vi "ret vs volt.vi"() -> ()   [LabVIEW 2014]
uses:
  <vilib>/Utility/file.llb/Write To Spreadsheet File (DBL).vi
  <vilib>/Analysis/NI_AALBase.lvlib
panel:
  out "min beam":dbl[](array[numeric])
  in  "LCVR temp":sgl=30.0 min=10 max=50
  out "max beam":dbl[](array[numeric])
  in  "Start calibration":bool
  out "Intensity Graph":dbl[][](graph)
  out "Horizontal ?":bool
  in  "OK":bool
  out "X - centroid":dbl[](array[numeric])
  out "Y - centroid":dbl[](array[numeric])
  in  "OpenStructureIn":T1={"Size"=88, "InterfaceType"=1, "Camera Number"=0, "CameraNumAtInterface"=0, "OpenFlags"=[], "OpenDWFlags"=[], "OpenPtrs"=[]} {"InterfaceType" items=["IEEE1394/FireWire", "IEEE1394/FireWire", "Matrox Helios CameraLink", "SiliconSoftware MicroEnableIII CL", "National Instruments CameraLink", "Gigabit Ethernet", "USB", "SiliconSoftware MicroEnable IV CL", "Reserved", "Reserved", "Generic CameraLink with CLSER.DLL"]}
  in  "Exposure in msec":u32
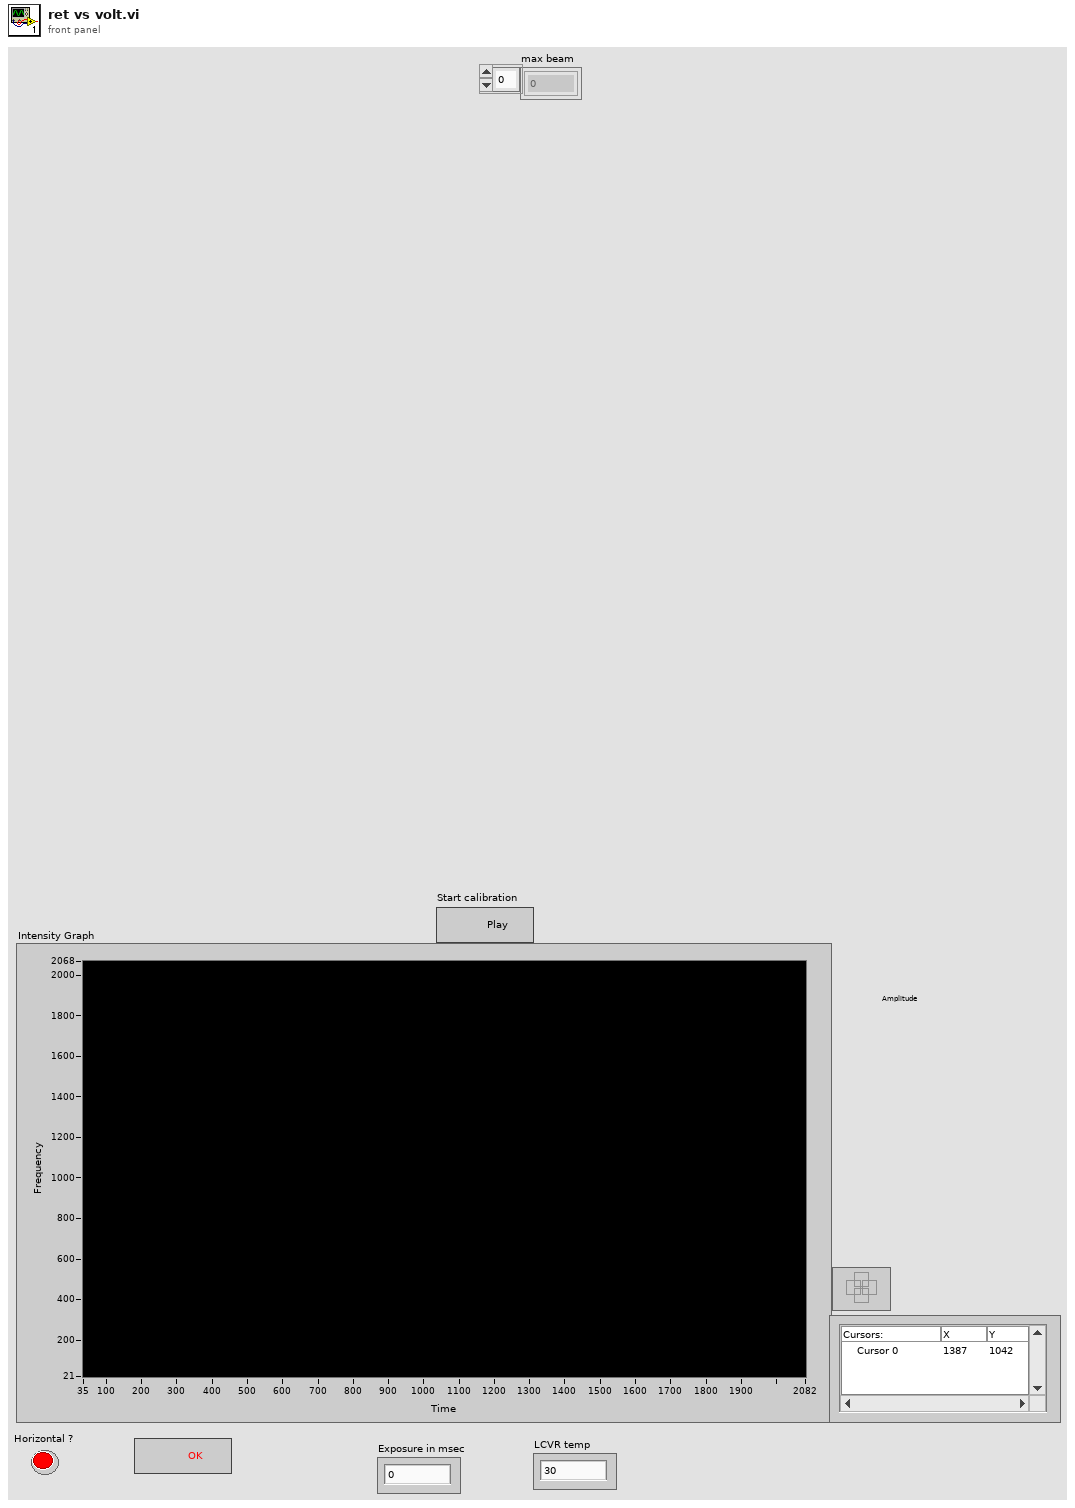
[diagram p1: front panel]
types:
  T1 = cluster{"Size":u16, "InterfaceType":u16, "Camera Number":u16, "CameraNumAtInterface":u16, "OpenFlags":u16[], "OpenDWFlags":u32[], "OpenPtrs":u32[]}
  T2 = cluster{"Device Handle":u32, "Pipe 0 Handle":u32, "Pipe 1 Handle":u32}[]
  T3 = cluster{"Device Handle":u32, "Pipe 0 Handle":u32, "Pipe 1 Handle":u32}
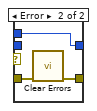
[diagram p2: hidden frame]
diagram:
  n1 = flat-sequence {
    tunnel: [w67] -> w58
    tunnel: [w66] -> w56
    tunnel: w58 -> [w112]
    tunnel: [w112] -> w57
    tunnel: w56 -> [w111]
    tunnel: [w111] -> w55
    tunnel: [w106] -> w28
    tunnel: w57 -> [w117]
    tunnel: w55 -> [w116]
    tunnel: [w114] -> w54
    tunnel: [w115] -> w52
    tunnel: w28 -> [w113]
    tunnel: [w113] -> w23
    tunnel: w54 -> [w173]
    tunnel: [w173] -> w53
    tunnel: w52 -> [w172]
    tunnel: [w172] -> w51
    tunnel: [w170] -> w24
    tunnel: w23 -> [w170]
    tunnel: w53 -> [w189]
    tunnel: w51 -> [w190]
    tunnel: [w183] -> w50
    tunnel: [w187] -> w47
    tunnel: [w186] -> w45
    tunnel: [w185] -> w41
    tunnel: [w184] -> w38
    tunnel: w29 -> [w183]
    tunnel: [w182] -> w25
    tunnel: w24 -> [w182]
    tunnel: [w176] -> w22
    tunnel: w50 -> [w253]
    tunnel: [w253] -> w49
    tunnel: [w250] -> w48
    tunnel: w47 -> [w250]
    tunnel: [w249] -> w46
    tunnel: w45 -> [w249]
    tunnel: [w248] -> w42
    tunnel: w41 -> [w248]
    tunnel: [w247] -> w39
    tunnel: w38 -> [w247]
    tunnel: [w246] -> w26
    tunnel: w25 -> [w246]
    tunnel: w22 -> [w245]
    tunnel: [w245] -> w20
    tunnel: w49 -> [w261]
    tunnel: [w261] -> w44
    tunnel: w48 -> [w255]
    tunnel: w46 -> [w257]
    tunnel: [w259] -> w43
    tunnel: w42 -> [w259]
    tunnel: [w258] -> w40
    tunnel: w39 -> [w258]
    tunnel: [w257] -> w35
    tunnel: [w256] -> w27
    tunnel: w26 -> [w256]
    tunnel: [w255] -> w21
    tunnel: w20 -> [w254]
    tunnel: [w254] -> w19
    tunnel: w44 -> [w265]
    tunnel: [w265] -> w18
    tunnel: w43 -> [w262]
    tunnel: w40 -> [w271]
    tunnel: [w270] -> w17
    tunnel: [w269] -> w16
    tunnel: [w268] -> w15
    tunnel: w35 -> [w268]
    tunnel: w27 -> [w267]
    tunnel: w21 -> [w264]
    tunnel: w19 -> [w263]
    tunnel: w18 -> [w327]
    tunnel: [w327] -> w14
    tunnel: w17 -> [w326]
    tunnel: [w326] -> w13
    tunnel: w16 -> [w325]
    tunnel: [w325] -> w12
    tunnel: w15 -> [w324]
    tunnel: [w324] -> w11
    tunnel: w14 -> [w337]
    tunnel: [w337] -> w10
    tunnel: w13 -> [w332]
    tunnel: [w330] -> w8
    tunnel: w12 -> [w333]
    tunnel: [w331] -> w6
    tunnel: w11 -> [w336]
    tunnel: [w336] -> w4
    tunnel: [w328] -> w2
    tunnel: w10 -> [w344]
    tunnel: [w344] -> w9
    tunnel: w8 -> [w343]
    tunnel: [w343] -> w7
    tunnel: w6 -> [w342]
    tunnel: [w342] -> w5
    tunnel: w4 -> [w341]
    tunnel: [w341] -> w3
    tunnel: w2 -> [w340]
    tunnel: [w340] -> w1
    tunnel: w9 -> [w357]
    tunnel: w7 -> [w352]
    tunnel: w5 -> [w351]
    tunnel: [w349] -> w37
    tunnel: [w348] -> w36
    tunnel: w3 -> [w348]
    tunnel: [w347] -> w34
    tunnel: [w346] -> w33
    tunnel: w1 -> [w345]
    tunnel: w37 -> [w412]
    tunnel: w36 -> [w427]
    tunnel: w34 -> [w418]
    tunnel: w33 -> [w417]
    frame #0 {
      w70 = u16 1 items=["Stop", "Run"] ("RecordingState")
      w73 = u16 1 items=["Auto", "Software", "External sequence start ", "External exposure control"] ("TriggerMode")
      w82 = u16 2 items=["nanoseconds", "microseconds", "milliseconds"] ("ExposureTimeBase")
      w61 = u32 8388608 ("Size")
      w92 = u16 0 items=["Stop", "Run"] ("RecordingState")
      n2 = local read "OpenStructureIn"() -> (w100:T1)
      n3 = Bundle By Name(cluster=w100, "InterfaceType"=u16 6) -> (w98:T1)
      n4 = call <userlib>:"OpenCameraEx.vi"("OpenStructureIn"=w98) -> ("error out"=w96:errorcluster, "hout"=w97:u64)  [unwired: 3 in, 2 out]
      n5 = call <userlib>:"CancelImages.vi"("error in (no error)"=w96, "ph"=w97) -> ()  [unwired: 1 in, 3 out]
      n6 = call <userlib>:"InitLibrary.vi"("error in (no error)"=w96, "InterfaceType"=u32 3, "ph"=w97) -> ("error out"=w93:errorcluster, "hout"=w94:u64)  [unwired: 7 in]
      n7 = call <userlib>:"SetBitAlignment.vi"("error in (no error)"=w93, "BitAlignent"=TRUE, "ph"=w94) -> ("error out"=w72:errorcluster, "hout"=w77:u64)  [unwired: 2 in, 1 out]
      n8 = call <userlib>:"SetStorageMode.vi"("error in (no error)"=w72, "StorageMode"=TRUE, "ph"=w77) -> ("error out"=w74:errorcluster, "hout"=w75:u64)  [unwired: 2 in, 1 out]
      n9 = call <userlib>:"SetTrigger.vi"("error in (no error)"=w74, "TriggerMode"=w73, "ph"=w75) -> ("error out"=w64:errorcluster, "hout"=w65:u64)  [unwired: 2 in, 1 out]
      n10 = call <userlib>:"AllocateBuffer.vi"("error in (no error)"=w64, "Size"=w61, "BufNr"=i16 -1, "ph"=w65) -> ("error out"=w63:errorcluster, "BufNrOut"=w59:i16, "hout"=w62:u64)  [unwired: 2 in, 3 out]
      n11 = call <userlib>:"SetRecordingState.vi"("ErrorIn"=w63, "RecordingState"=w92, "ph"=w62) -> ("ErrorOut"=w90:errorcluster, "hout"=w91:u64)  [unwired: 2 in, 1 out]
      n12 = case shown="No Error" w90 {
        tunnel: [w102 w104] -> w88
        tunnel: w90 -> [w102 w105]
        tunnel: w91 -> [w101 _]
        tunnel: [w101 w103] -> w89
        tunnel: w77 -> [_ w103]
        frame No Error {
        }
        frame Error {
          n13 = call <vilib>:"Clear Errors.vi"("error in (no error)"=w105) -> ("error out"=w104:errorcluster)  [unwired: 5 in, 1 out]
        }
      }
      n14 = call <userlib>:"AllocateBuffer.vi"("error in (no error)"=w88, "Size"=w61, "BufNr"=i16 -1, "ph"=w89) -> ("error out"=w85:errorcluster, "hout"=w86:u64)  [unwired: 2 in, 4 out]
      n15 = call <userlib>:"SetDelayExposureTime.vi"("ph"=w86, "Delay"=u32 0, "Exposure"="Exposure in msec", "error in (no error)"=w85, "DelayTimeBase"=w82, "ExposureTimeBase"=w82) -> ("hout"=w81:u64, "error out"=w80:errorcluster)  [unwired: 7 in, 1 out]
      n16 = call <userlib>:"ArmCamera.vi"("error in (no error)"=w80, "ph"=w81) -> ("error out"=w78:errorcluster, "hout"=w79:u64)  [unwired: 2 out]
      n17 = call <userlib>:"AllocateBuffer.vi"("error in (no error)"=w78, "Size"=w61, "BufNr"=w59, "ph"=w79) -> ("error out"=w68:errorcluster, "hout"=w71:u64)  [unwired: 2 in, 4 out]
      n18 = call <userlib>:"SetRecordingState.vi"("ErrorIn"=w68, "RecordingState"=w70, "ph"=w71) -> ("ErrorOut"=w66:errorcluster, "hout"=w67:u64)  [unwired: 2 in, 1 out]
    }
    frame #1 {
      n19 = One Button Dialog(message="After starting and making the beam\nhorizintal cross one of the beam with\npolariser place lcvr and then press OK\n button to initiate voltage vs ret \n   calibration              ", button name ("OK")="Got it !!") -> ()  [unwired: 1 out]
      n20 = call "File Dialog3"("prompt"="Select folder containing matlab files for execution") -> ("selected path"=w107:path)  [unwired: 11 in, 3 out]
      n21 = Path To String(path=w107) -> (string=w106:string)
    }
    frame #2 {
      # "To check if  beams of beam splitter are perfectly horizontal"
      n22 = while {
        tunnel: ["Start calibration"] -> w118
        stop <- "Start calibration" stop-if-true
      }
      n23 = while {
        shift-right: [w125] -> w115
        shift-left: w117 -> [w131]
        shift-right: [w124] -> w114
        shift-left: w116 -> [w130]
        stop <- w120 stop-if-true
        n24 = call <userlib>:"ForceTrigger.vi"("ph"=w131, "error in (no error)"=w130) -> ("hout"=w129:u64, "error out"=w128:errorcluster)  [unwired: 1 in, 2 out]
        n25 = call "grab image_2.vi"("ErrorIn"=w128, "Image number"=u32 0, "BuffNr"=i16 0, "ph"=w129) -> ("output image"=→"Intensity Graph":dbl[][], "error out"=w124:errorcluster, "Buffer_Ready"=w121:bool, "hout"=w125:u64)  [unwired: 4 in]
        n26 = local read "OK"() -> (w122:bool)
        n27 = And(x=w121, y=w122) -> (x .and. y?=w120:bool)
      }
      n28 = case shown="True" w118 {
        tunnel: w113 -> [_ w132]
        frame False {
        }
        frame True {
          n29 = while {
            tunnel: w132 -> [w134]
            stop <- w133 stop-if-true
            n30 = flat-sequence {
              tunnel: w134 -> [w141]
              tunnel: [w151] -> w133
              frame #0 {
                n31 = local read "Intensity Graph"() -> (w135:dbl[][])
                n32 = property on="Intensity Graph" class="IntGraph (strict)"() -> ("Cursor.Cursor X"=w142:dbl)  [unwired: 2 in, 2 out]
                n33 = script code="cd(path);\n[ax,ay]=calib1(da,s);\nx=[ax(1),ay(1)];\ny=[ax(2),ay(2)];"("path"=w141, "da"=w135, "s"=w142) -> ("x"=w140:dbl[], "y"=w139:dbl[])  [unwired: 1 in, 1 out]
                "X - centroid" <- w140
                "Y - centroid" <- w139
                n34 = Reshape Array(w135, 4194304 ("dimension size")) -> (w143:dbl[])
                n35 = call <vilib>:"Median.vi"("X"=w143) -> ("median"=w138:dbl)  [unwired: 1 out]
                n36 = Index Array(array=w140, index=1) -> (element=w148:dbl)
                n37 = Index Array(array=w139, index=1) -> (element=w147:dbl)
                n38 = call "= to within Tolerance"("Operand 2"=w147, "Operand 1"=w148) -> ("Result"=w146:dynamicdata)  [unwired: 8 in, 1 out]
                n39 = Add(x=w138, y=700.0) -> (x+y=w136:dbl)
                n40 = call "Convert from Dynamic Data"("Dynamic Data Type"=w146) -> ("Scalar"=→"Horizontal ?":bool)  [unwired: 3 in]
                n41 = property on="Intensity Graph" class="IntGraph (strict)"("ZScale.Maximum"=w136) -> ()  [unwired: 2 in, 2 out]
              }
              frame #1 {
                n42 = Two Button Dialog(message="repeat curve \n  fit?         ", 1:"yes" ("F button name (\"Cancel\")"), 2:"no" ("T button name (\"OK\")")) -> (T button?=w151:bool)
                n43 = local write "OK"(w151) -> ()
              }
            }
          }
        }
      }
    }
    frame #3 {
      n44 = local read "X - centroid"() -> (w162:dbl[])
      n45 = local read "Y - centroid"() -> (w161:dbl[])
      n46 = local write "OK"(FALSE ("OK")) -> ()
      n47 = local read "Intensity Graph"() -> (w171:dbl[][])
      n48 = call "Convert to Dynamic Data3"("Array"=w161) -> ("Dynamic Data Type"=w160:dynamicdata)  [unwired: 3 in]
      n49 = call "Convert to Dynamic Data2"("Array"=w162) -> ("Dynamic Data Type"=w157:dynamicdata)  [unwired: 3 in]
      n50 = call "Convert from Dynamic Data3"("Dynamic Data Type"=w160) -> ("Scalar"=w159:dbl)  [unwired: 3 in]
      n51 = call "Convert from Dynamic Data4"("Dynamic Data Type"=w160) -> ("Scalar"=w158:dbl)  [unwired: 3 in]
      n52 = call "Convert from Dynamic Data5"("Dynamic Data Type"=w157) -> ("Scalar"=w156:dbl)  [unwired: 3 in]
      n53 = call "Convert from Dynamic Data6"("Dynamic Data Type"=w157) -> ("Scalar"=w155:dbl)  [unwired: 3 in]
      n54 = Index Array(array=w171, index (row)=w159, index (col)=w158) -> (element=w164:dbl)
      n55 = Index Array(array=w171, index (row)=w156, index (col)=w155) -> (element=w165:dbl)
      n56 = Greater?(x=w164, y=w165) -> (0:w163:bool)
      n57 = Greater?(x=w165, y=w164) -> (0:w168:bool)
      n58 = Select(t=w162, s=w163, f=w161) -> (s? t:f=→"min beam":dbl[])
      n59 = Select(t=w162, s=w168, f=w161) -> (s? t:f=→"max beam":dbl[])
    }
    frame #4 {
      w181 = dbl[] []
      # "to get beams of nearly equal intensity\nfor curve fitting in matlab. Note this \nvoltage neednot correspond to 90deg\nnor might it give good intensity values \nfor curve fit after aligning the lcvr"
      # "to get volt corresponding to 180deg ret"
      n60 = call "version.vi"("USB Open Device Cluster"=w183) -> ("Version"=w187:dbl)  [unwired: 10 in]
      n61 = for {
        N: 100 -> [_]
        tunnel: w183 -> [w208]
        shift-right: [w205] -> w177
        shift-left: w181 -> [w206]
        shift-right: [w203] -> w185
        shift-left: w190 -> [w204]
        shift-right: [w201] -> w184
        shift-left: w189 -> [w202]
        shift-right: [w200] -> w180
        shift-left: w181 -> [w199]
        tunnel: w187 -> [w194]
        shift-right: [w193] -> w179
        shift-left: w181 -> [w192]
        i -> [w207]
        n62 = flat-sequence {
          tunnel: w208 -> [w239]
          tunnel: w207 -> [w237]
          tunnel: w206 -> [w234]
          tunnel: w204 -> [w228]
          tunnel: w202 -> [w226]
          tunnel: w199 -> [w221]
          tunnel: [w233] -> w198
          tunnel: [w227] -> w197
          tunnel: [w225] -> w196
          tunnel: [w222] -> w195
          tunnel: w194 -> [w220]
          tunnel: [w216] -> w193
          tunnel: w192 -> [w215]
          tunnel: [w241] -> w200
          tunnel: [w242] -> w201
          tunnel: [w243] -> w203
          tunnel: [w244] -> w205
          tunnel: w198 -> [w244]
          tunnel: w197 -> [w243]
          tunnel: w196 -> [w242]
          tunnel: w195 -> [w241]
          frame #0 {
            n63 = call <userlib>:"ForceTrigger.vi"("ph"=w228, "error in (no error)"=w226) -> ("hout"=w232:u64, "error out"=w231:errorcluster)  [unwired: 1 in, 2 out]
            n64 = Divide(x=w237, y=10) -> (x/y=w235:dbl)
            n65 = local read "max beam"() -> (w224:dbl[])
            n66 = local read "min beam"() -> (w219:dbl[])
            n67 = call "Meadowlark USB Set Voltage.VI"("LC Voltage"=w235, "LC Channel"=1, "FW Version"=w220, "USB Open Device Cluster"=w239) -> ()  [unwired: 1 out]
            n68 = Build Array (concatenate)(w234, w235) -> (w233:dbl[])
            n69 = call "grab image_2.vi"("ErrorIn"=w231, "Image number"=u32 0, "BuffNr"=i16 0, "ph"=w232) -> ("output image"=w218:dbl[][], "error out"=w225:errorcluster, "hout"=w227:u64)  [unwired: 4 in, 1 out]
            n70 = call "Convert to Dynamic Data6"("Array"=w219) -> ("Dynamic Data Type"=w214:dynamicdata)  [unwired: 3 in]
            n71 = call "Convert to Dynamic Data"("Array"=w224) -> ("Dynamic Data Type"=w211:dynamicdata)  [unwired: 3 in]
            n72 = local write "Intensity Graph"(w218) -> ()
            n73 = call "Convert from Dynamic Data7"("Dynamic Data Type"=w214) -> ("Scalar"=w213:dbl)  [unwired: 3 in]
            n74 = call "Convert from Dynamic Data8"("Dynamic Data Type"=w214) -> ("Scalar"=w212:dbl)  [unwired: 3 in]
            n75 = call "Convert from Dynamic Data9"("Dynamic Data Type"=w211) -> ("Scalar"=w210:dbl)  [unwired: 3 in]
            n76 = call "Convert from Dynamic Data10"("Dynamic Data Type"=w211) -> ("Scalar"=w209:dbl)  [unwired: 3 in]
            n77 = Index Array(array=w218, index (row)=w213, index (col)=w212) -> (element=w217:dbl)
            n78 = Index Array(array=w218, index (row)=w210, index (col)=w209) -> (element=w223:dbl)
            n79 = Build Array (concatenate)(w221, w223) -> (w222:dbl[])
            n80 = Build Array (concatenate)(w215, w217) -> (w216:dbl[])
          }
          frame #1 {
            n81 = Wait (ms)(milliseconds to wait=u32 30) -> ()  [unwired: 1 out]
          }
        }
      }
      n82 = Subtract(x=w180, y=w179) -> (x-y=w175:dbl[])
      n83 = Array Max & Min(array=w180) -> (min index (indices)=w188:i32)  [unwired: 3 out]
      n84 = Absolute Value(x=w175) -> (abs(x)=w174:dbl[])
      n85 = Index Array(array=w177, index=w188) -> (element=w186:dbl)
      n86 = Array Max & Min(array=w174) -> (min index (indices)=w178:i32)  [unwired: 3 out]
      n87 = Index Array(array=w177, index=w178) -> (element=w176:dbl)
    }
    frame #5 {
      n88 = One Button Dialog(message="current retardance of lcvr \nis 180deg rotate lcvr to get\nthe beam which was crossed \nto maximum intensity then \nselect the split point on the \nimage using cursor and click OK. \nThis calculates the new position \nof the two beams.       ", button name ("OK")="Yes") -> ()  [unwired: 1 out]
    }
    frame #6 {
      n89 = call "Meadowlark USB Set Voltage.VI"("LC Voltage"=w257, "LC Channel"=1, "FW Version"=w255, "USB Open Device Cluster"=w261) -> ()  [unwired: 1 out]
    }
    frame #7 {
      n90 = flat-sequence {
        tunnel: w267 -> [w272]
        tunnel: [w272] -> w266
        tunnel: w266 -> [w283]
        tunnel: w265 -> [w278]
        tunnel: w264 -> [w277]
        tunnel: w263 -> [w275]
        tunnel: w262 -> [w274]
        frame #0 {
          n91 = while {
            stop <- w273 stop-if-true
            n92 = local read "OK"() -> (w273:bool)
          }
        }
        frame #1 {
          n93 = call "Meadowlark USB Set Voltage.VI"("LC Voltage"=w275, "LC Channel"=1, "FW Version"=w277, "USB Open Device Cluster"=w278) -> ()  [unwired: 1 out]
          n94 = Two Button Dialog(message="Recalibrate position\nof the beams?  ", 1:"No" ("F button name (\"Cancel\")"), 2:"Yes" ("T button name (\"OK\")")) -> (T button?=w279:bool)
          n95 = case shown="True" w279 {
            tunnel: w283 -> [_ w287]
            tunnel: w274 -> [_ w284]
            frame False {
            }
            frame True {
              n96 = flat-sequence {
                tunnel: w287 -> [w290]
                tunnel: [w290] -> w286
                tunnel: [w289] -> w285
                tunnel: w284 -> [w288]
                tunnel: w286 -> [w303]
                tunnel: w285 -> [w299]
                frame #0 {
                  n97 = while {
                    shift-right: [w293] -> _
                    shift-left: w288 -> [w292]
                    tunnel: [w291] -> w289
                    stop <- w298 stop-if-true
                    n98 = call <userlib>:"ForceTrigger.vi"("ph"=w292) -> ("hout"=w297:u64, "error out"=w294:errorcluster)  [unwired: 2 in, 2 out]
                    n99 = call "grab image_2.vi"("ErrorIn"=w294, "Image number"=u32 0, "BuffNr"=i16 0, "ph"=w297) -> ("output image"=w291:dbl[][], "hout"=w293:u64)  [unwired: 4 in, 2 out]
                    n100 = local write "Intensity Graph"(w291) -> ()
                    n101 = local read "OK"() -> (w298:bool)
                  }
                }
                frame #1 {
                  n102 = property on="Intensity Graph" class="IntGraph (strict)"() -> ("Cursor.Cursor X"=w302:dbl)  [unwired: 2 in, 2 out]
                  n103 = script code="cd(path);\n[ax,ay]=calib1(da,s);\nx=[ax(1),ay(1)];\ny=[ax(2),ay(2)];"("path"=w303, "da"=w299, "s"=w302) -> ("x"=w301:dbl[], "y"=w300:dbl[])  [unwired: 1 in, 1 out]
                  n104 = local write "X - centroid"(w301) -> ()
                  n105 = local write "Y - centroid"(w300) -> ()
                  n106 = Index Array(array=w301, index=1) -> (element=w307:dbl)
                  n107 = Index Array(array=w300, index=1) -> (element=w306:dbl)
                  n108 = call "= to within Tolerance2"("Operand 2"=w306, "Operand 1"=w307) -> ("Result"=w305:dynamicdata)  [unwired: 8 in, 1 out]
                  n109 = call "Convert from Dynamic Data2"("Dynamic Data Type"=w305) -> ("Scalar"=w304:bool)  [unwired: 3 in]
                  n110 = local write "Horizontal ?"(w304) -> ()
                }
              }
            }
          }
        }
      }
      n111 = while {
        shift-right: [w315] -> w270
        shift-left: w262 -> [w321]
        shift-right: [w314] -> w269
        shift-left: w271 -> [w320]
        stop <- w311 stop-if-true
        n112 = call <userlib>:"ForceTrigger.vi"("ph"=w321, "error in (no error)"=w320) -> ("hout"=w319:u64, "error out"=w318:errorcluster)  [unwired: 1 in, 2 out]
        n113 = call "grab image_2.vi"("ErrorIn"=w318, "Image number"=u32 0, "BuffNr"=i16 0, "ph"=w319) -> ("output image"=w310:dbl[][], "error out"=w314:errorcluster, "Buffer_Ready"=w312:bool, "hout"=w315:u64)  [unwired: 4 in]
        n114 = local read "OK"() -> (w313:bool)
        n115 = local write "Intensity Graph"(w310) -> ()
        n116 = And(x=w312, y=w313) -> (x .and. y?=w311:bool)
      }
    }
    frame #8 {
      n117 = One Button Dialog(message="Now we will record background so \nswitch off the source and prees \nOK button                ", button name ("OK")="OK") -> ()  [unwired: 1 out]
    }
    frame #9 {
      w329 = i16 0 ("BuffNr")
      n118 = call <userlib>:"ForceTrigger.vi"("ph"=w332, "error in (no error)"=w333) -> ("hout"=w335:u64, "error out"=w334:errorcluster)  [unwired: 1 in, 2 out]
      n119 = call "grab image_2.vi"("ErrorIn"=w334, "Image number"=w329, "BuffNr"=w329, "ph"=w335) -> ("output image"=w328:dbl[][], "error out"=w331:errorcluster, "hout"=w330:u64)  [unwired: 4 in, 1 out]
      n120 = local write "Intensity Graph"(w328) -> ()
    }
    frame #10 {
      n121 = One Button Dialog(message="Switch on source\nto perform volt vs\nret calibration and\npress OK     ", button name ("OK")="OK") -> ()  [unwired: 1 out]
    }
    frame #11 {
      w350 = dbl[] []
      n122 = call "version.vi"("USB Open Device Cluster"=w357) -> ("Version"=w356:dbl)  [unwired: 10 in]
      n123 = script code="clear all"() -> ()  [unwired: 1 in, 1 out]
      n124 = for {
        N: 100 -> [_]
        tunnel: w357 -> [w374]
        shift-right: [w372] -> w347
        shift-left: w352 -> [w370]
        shift-right: [w371] -> w346
        shift-left: w351 -> [w369]
        tunnel: w356 -> [w368]
        shift-right: [w365] -> w355
        shift-left: w350 -> [w364]
        shift-right: [w363] -> w354
        shift-left: w350 -> [w361]
        shift-right: [w362] -> w353
        shift-left: w350 -> [w360]
        tunnel: w345 -> [w359]
        i -> [w373]
        n125 = flat-sequence {
          tunnel: w374 -> [w380]
          tunnel: w373 -> [w378]
          tunnel: w368 -> [w376]
          tunnel: [w375] -> w366
          tunnel: [w381] -> w367
          tunnel: w366 -> [w381]
          tunnel: [w406] -> w372
          tunnel: [w405] -> w371
          tunnel: w370 -> [w404]
          tunnel: w369 -> [w403]
          tunnel: w367 -> [w400]
          tunnel: [w399] -> w365
          tunnel: w364 -> [w398]
          tunnel: [w395] -> w363
          tunnel: [w394] -> w362
          tunnel: w361 -> [w393]
          tunnel: w360 -> [w392]
          tunnel: w359 -> [w383]
          frame #0 {
            n126 = Divide(x=w378, y=10) -> (x/y=w375:dbl)
            n127 = call "Meadowlark USB Set Voltage.VI"("LC Voltage"=w375, "LC Channel"=1, "FW Version"=w376, "USB Open Device Cluster"=w380) -> ()  [unwired: 1 out]
          }
          frame #1 {
            n128 = Wait (ms)(milliseconds to wait=u32 30) -> ()  [unwired: 1 out]
          }
          frame #2 {
            n129 = Build Array (concatenate)(w398, w400) -> (w399:dbl[])
            n130 = call <userlib>:"ForceTrigger.vi"("ph"=w404, "error in (no error)"=w403) -> ("hout"=w410:u64, "error out"=w409:errorcluster)  [unwired: 1 in, 2 out]
            n131 = local read "X - centroid"() -> (w402:dbl[])
            n132 = local read "Y - centroid"() -> (w401:dbl[])
            n133 = call "grab image_2.vi"("ErrorIn"=w409, "Image number"=u32 0, "BuffNr"=i16 0, "ph"=w410) -> ("output image"=w385:dbl[][], "error out"=w405:errorcluster, "hout"=w406:u64)  [unwired: 4 in, 1 out]
            n134 = Subtract(x=w385, y=w383) -> (x-y=w384:dbl[][])
            n135 = call "Convert to Dynamic Data4"("Array"=w402) -> ("Dynamic Data Type"=w391:dynamicdata)  [unwired: 3 in]
            n136 = call "Convert to Dynamic Data5"("Array"=w401) -> ("Dynamic Data Type"=w388:dynamicdata)  [unwired: 3 in]
            n137 = call "Convert from Dynamic Data11"("Dynamic Data Type"=w391) -> ("Scalar"=w390:dbl)  [unwired: 3 in]
            n138 = call "Convert from Dynamic Data12"("Dynamic Data Type"=w391) -> ("Scalar"=w389:dbl)  [unwired: 3 in]
            n139 = call "Convert from Dynamic Data13"("Dynamic Data Type"=w388) -> ("Scalar"=w387:dbl)  [unwired: 3 in]
            n140 = call "Convert from Dynamic Data14"("Dynamic Data Type"=w388) -> ("Scalar"=w386:dbl)  [unwired: 3 in]
            n141 = local write "Intensity Graph"(w384) -> ()
            n142 = Index Array(array=w384, index (row)=w390, index (col)=w389) -> (element=w397:dbl)
            n143 = Index Array(array=w384, index (row)=w387, index (col)=w386) -> (element=w396:dbl)
            n144 = Build Array (concatenate)(w393, w397) -> (w395:dbl[])
            n145 = Build Array (concatenate)(w392, w396) -> (w394:dbl[])
          }
        }
      }
      n146 = Build Array(w355, w354, w353) -> (w349:dbl[][])
    }
    frame #12 {
      # "If matlab dosn't give proper o/p then jst transpose the matrix\ncoz labview takes 1D array as 1-row n-columns but matlab o/p might be \nn-row 1-column. Thus transposing the matrix eliminates this issue. Also \ndont forget to clear all variables else ur o/p will be nasty due to stray variables"
      n147 = call <userlib>:"CancelImages.vi"("error in (no error)"=w417, "ph"=w418) -> ("error out"=w419:errorcluster, "hout"=w420:u64)  [unwired: 1 in, 1 out]
      n148 = call <userlib>:"Cleanup.vi"("error in (no error)"=w419, "ph"=w420) -> ("error out"=w422:errorcluster, "hout"=w421:u64)  [unwired: 8 in]
      n149 = call <userlib>:"CloseCamera.vi"("ErrorIn"=w422, "Handle in"=w421) -> ()  [unwired: 1 in, 3 out]
      n150 = call "File Dialog"("prompt"="select folder which contains\nmatlab script of volt vs ret") -> ("selected path"=w411:path)  [unwired: 11 in, 3 out]
      n151 = script code="cd(pat);\n[ret,volt]=volt_vs_ret(arr,v);\nret=ret';\nvolt=volt';"("pat"=w411, "arr"=w412, "v"=w427) -> ("ret"=w415:dbl[], "volt"=w414:dbl[])  [unwired: 1 in, 1 out]
      n152 = call "File Dialog2"("prompt"="select folder to store volt vs ret data") -> ("selected path"=w425:path)  [unwired: 11 in, 3 out]
      n153 = Build Array(w415, w414) -> (w416:dbl[][])
      n154 = call-poly <vilib>:"Write To Spreadsheet File.vi"("delimiter (\\t)"="," ("delimiter (\\t)"), "transpose? (no:F)"=FALSE, "2D data"=w416, "file path (dialog if empty)"=w425) -> ()  [unwired: 4 in, 1 out]
    }
  }
  n155 = call "Meadowlark USB Easy Open.vi"() -> ("USB Device and Pipes Array"=w31:T2)  [unwired: 2 out]
  n156 = Index Array(array=w31, index=0) -> (element=w29:T3)
  n157 = call "Set temp.vi"("Temp"="LCVR temp", "USB Open Device Cluster"=w29) -> ()  [unwired: 1 in]
